vi "sub_Create_Packet_Header.vi"(1 "Packet Number":i32) -> (0 "header bits":i8[](array[numeric]))   [LabVIEW 2022 SP3]
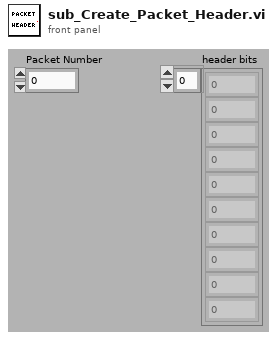
[diagram p1: front panel]
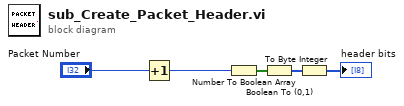
[diagram p0: block diagram]
diagram:
  n1 = Increment(x="Packet Number") -> (x+1=w1:i32)
  n2 = Number To Boolean Array(number=w1) -> (Boolean array=w3:bool[])
  n3 = Boolean To (0,1)(Boolean=w3) -> (0, 1=w4:i16[])
  n4 = To Byte Integer(number=w4) -> (8bit integer=→"header bits":i8[])
